vi "Read B.vi"(8 "error in (no error)":errorcluster, 11 "Add in":refnum<class "Add.lvclass">) -> (0 "error out":errorcluster, 2 "B":dbl, 3 "Add out":refnum<class "Add.lvclass">)   [LabVIEW 2023, in "Add.lvclass"]
uses:
  Add.lvclass
  Add.lvclass/Add.ctl
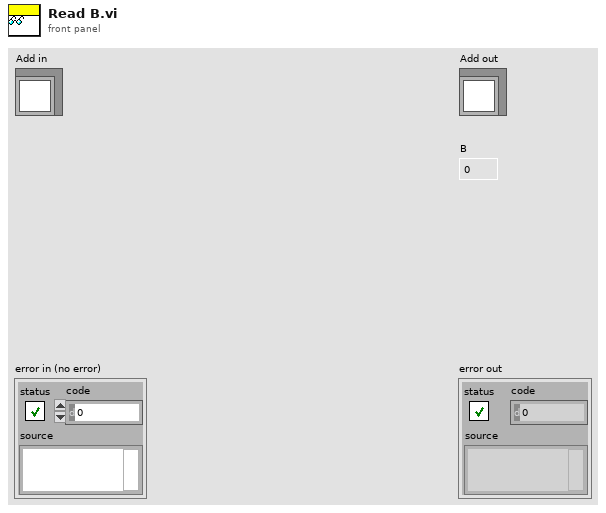
[diagram p1: front panel]
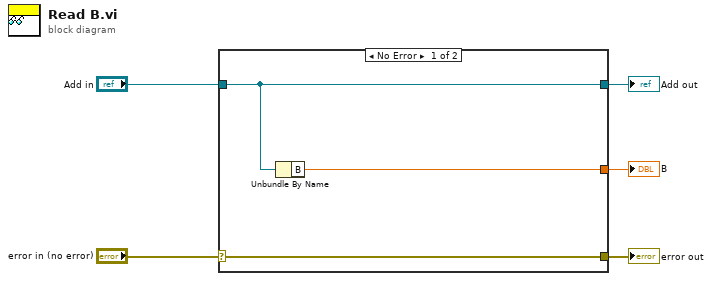
[diagram p0: block diagram]
diagram:
  n1 = case shown="No Error" "error in (no error)" {
    selector: "error in (no error)" -> [w8 w9]
    tunnel: [w8 w9] -> w4
    tunnel: [w7 w10] -> w2
    tunnel: "Add in" -> [w7 w10]
    tunnel: [w6 _] -> w1
    frame No Error {
      n2 = Unbundle By Name(w7) -> ("B"=w6:dbl)
    }
    frame Error {
    }
  }
  "error out" <- w4
  "Add out" <- w2
  "B" <- w1
